vi "Read Network Slave.vi"(8 "error in (no error)":errorcluster, 11 "Modbus slave in":refnum<class "Modbus Slave.lvclass">) -> (0 "error out":errorcluster, 2 "network slave":refnum<class "Network Slave.lvclass">, 3 "Modbus slave out":refnum<class "Modbus Slave.lvclass">)   [LabVIEW 2020, in "Modbus Slave.lvclass"]
doc: "This VI is an accessor for the <B>network slave</B> stored in the Modbus slave instance. This accessor can be used as a property node. This network slave is used by the Modbus instance to communicate on the physical bus."
uses:
  <vilib>/Modbus/slave/Modbus Slave.lvclass
  <vilib>/Modbus/subvis/Protocol/Interfaces/Network Slave/Network Slave.lvclass
  <vilib>/Modbus/slave/Modbus Slave.lvclass/Modbus Slave.ctl
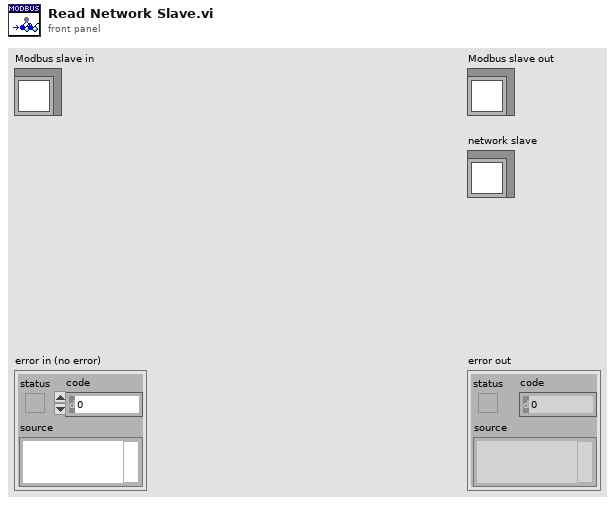
[diagram p1: front panel]
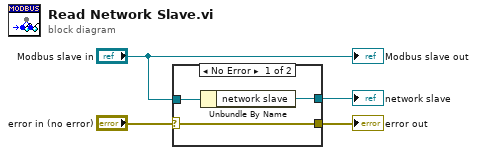
[diagram p0: block diagram]
diagram:
  n1 = case shown="No Error" "error in (no error)" {
    selector: "error in (no error)" -> [w5 w8]
    tunnel: "Modbus slave in" -> [w7 _]
    tunnel: [w6 _] -> w3
    tunnel: [w5 w8] -> w1
    frame No Error {
      n2 = Unbundle By Name(w7) -> ("network slave"=w6:refnum<class "Network Slave.lvclass">)
    }
    frame Error {
    }
  }
  "error out" <- w1
  "network slave" <- w3
  "Modbus slave out" <- "Modbus slave in"
